vi "Use memory.vi"(5 "memory allocated for LabVIEW":u64) -> (2 "Used memory":string)   [LabVIEW 2020]
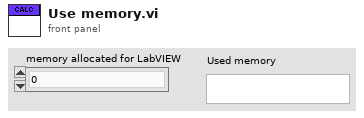
[diagram p1: front panel]
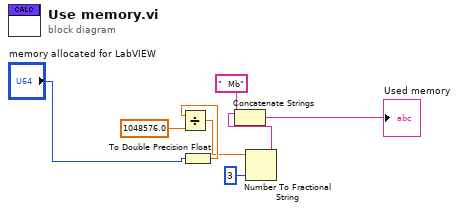
[diagram p0: block diagram]
diagram:
  n1 = To Double Precision Float(number="memory allocated for LabVIEW") -> (double precision float=w8:dbl)
  n2 = Divide(x=w8, y=1048576.0) -> (x/y=w6:dbl)
  n3 = Number To Fractional String(number=w6, precision (6)=i16 3) -> (F-format string=w5:string)  [unwired: 2 in]
  n4 = Concatenate Strings(w5, "  Mb" ("string")) -> (→"Used memory":string)
